vi "FRCts20_Backend_FGVDequeueDataReturn.vi"(6 "Engine_Refnums":T1, 7 "Operation":T4, 8 "error in (no error)":errorcluster) -> (0 "error out":errorcluster, 1 "Key":string, 2 "Message Value":string, 3 "Message Name":string, 4 "Engine_Refnums Out":T1)   [LabVIEW 2013, in "FRCts20_Backend_Engine.lvlib"]
doc: "Takes the AMC queues and lets us dequeue data. All it stores is the AMC queues."
uses:
  FRCts20_Backend_Engine.lvlib
  FRCts20_Backend_EngineRefnums.ctl
  INI_Accessor/FRCts20_Backend_INI Controller.lvclass
  Dependencies/AMC/_SubVIs/TypeDefs/Message Queue.ctl
  Dependencies/AMC/_SubVIs/TypeDefs/Message.ctl
  Dependencies/Keyed Array/KeyedArray.ctl
  <vilib>/addons/database/Connection.llb/Conn ObjectReference.ctl
  FRCts20_Backend_DequeueDataOperations.ctl
  Dependencies/AMC/AMC.lvlib
  Dependencies/Keyed Array/Tools_KeyedArray.lvlib
  <vilib>/addons/database/NI_Database_API.lvlib
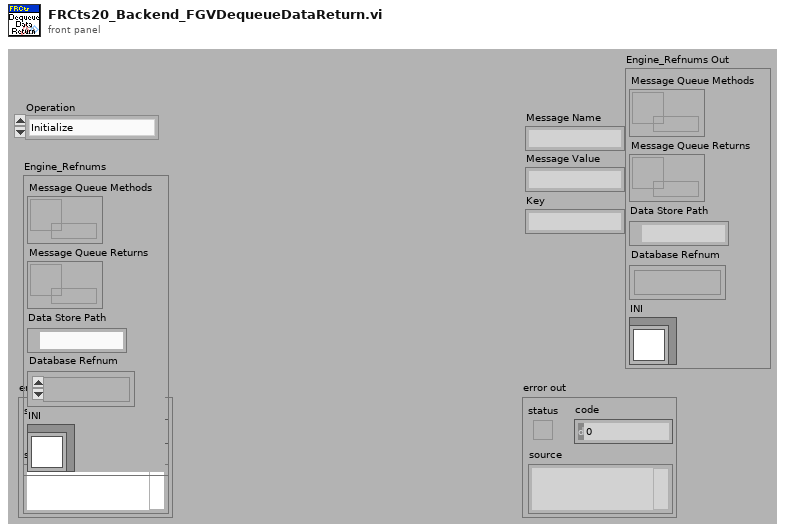
[diagram p1: front panel]
types:
  T1 = typedef "FRCts20_Backend_Engine.lvlib/FRCts20_Backend_EngineRefnums.ctl" = cluster{"Message Queue Methods":T2, "Message Queue Returns":T2, "Data Store Path":path, "Database Refnum":T3, "INI":refnum<class "FRCts20_Backend_INI Controller.lvclass">}
  T2 = typedef "AMC.lvlib/Message Queue.ctl" = refnum<queue>
  T3 = typedef "NI_Database_API.lvlib/Conn ObjectReference.ctl" = refnum<k1>
  T4 = typedef "FRCts20_Backend_Engine.lvlib/FRCts20_Backend_DequeueDataOperations.ctl" = enum16{"Initialize", "DequeueDataReturn", "GetQueues"}
  T5 = typedef "Tools_KeyedArray.lvlib/KeyedArray.ctl" = cluster{"keys":string[], "values":string[]}
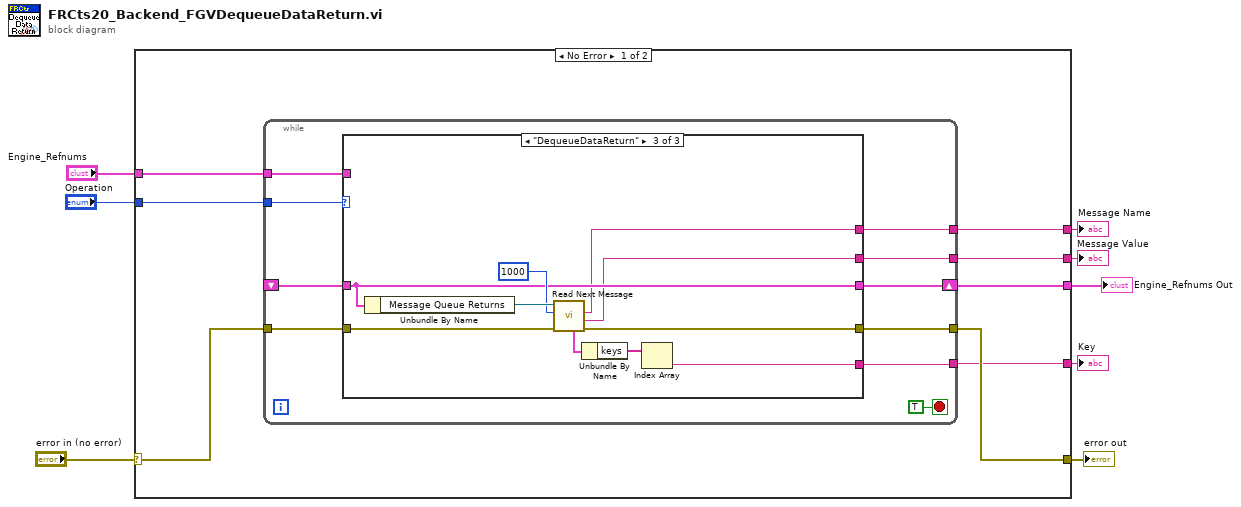
[diagram p0: block diagram]
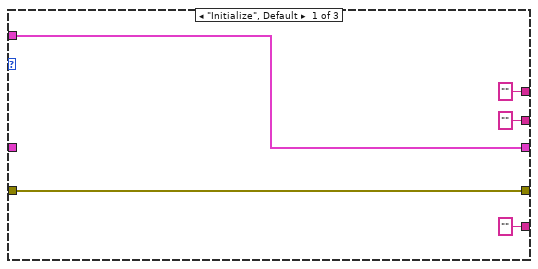
[diagram p2: hidden frame]
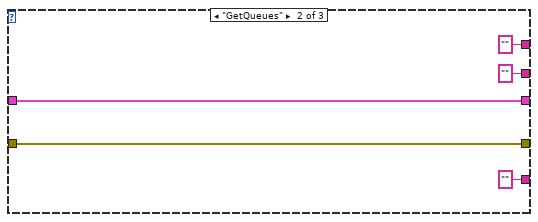
[diagram p3: hidden frame]
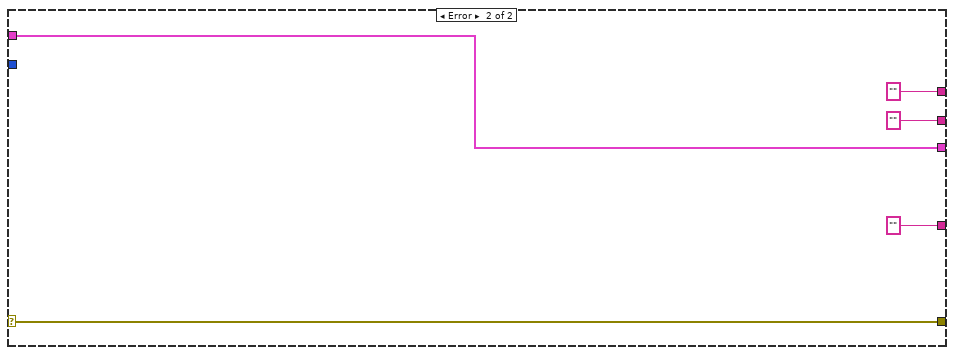
[diagram p4: hidden frame]
diagram:
  n1 = case shown="No Error" "error in (no error)" {
    selector: "error in (no error)" -> [w14 w51]
    tunnel: [w16 w51] -> w7
    tunnel: "Engine_Refnums" -> [w15 w47]
    tunnel: "Operation" -> [w13 _]
    tunnel: [w12 "" ("Message Name")] -> w4
    tunnel: [w11 "" ("Message Value")] -> w3
    tunnel: [w10 "" ("String")] -> w2
    tunnel: [w9 w47] -> w1
    frame No Error {
      n2 = while {
        tunnel: [w25] -> w16
        tunnel: w15 -> [w24]
        shift-right: [w23] -> w9
        shift-left: _ -> [w22]
        tunnel: w14 -> [w21]
        tunnel: w13 -> [w20]
        tunnel: [w19] -> w12
        tunnel: [w18] -> w11
        tunnel: [w17] -> w10
        stop <- TRUE stop-if-true
        n3 = case shown="\"DequeueDataReturn\"" w20 {
          tunnel: [w30 w36 w42] -> w25
          tunnel: w24 -> [w31 _ _]
          tunnel: [w31 w32 w43] -> w23
          tunnel: w22 -> [_ w32 w43]
          tunnel: w21 -> [w30 w36 w45]
          tunnel: ["" ("Message Name") "" ("Message Name") w41] -> w19
          tunnel: ["" ("Message Value") "" ("Message Value") w40] -> w18
          tunnel: ["" ("String") "" ("String") w37] -> w17
          frame "Initialize", Default {
          }
          frame "GetQueues" {
          }
          frame "DequeueDataReturn" {
            n4 = Unbundle By Name(w43) -> ("Message Queue Returns"=w46:T2)
            n5 = call "Read Next Message.vi"("error in (no error)"=w45, "timeout (1ms)"=1000, "Message Queue in"=w46) -> ("error out"=w42:errorcluster, "Message Value"=w40:string, "Message Name"=w41:string, "Message Attributes"=w39:T5)  [unwired: 2 in, 3 out]
            n6 = Unbundle By Name(w39) -> ("keys"=w38:string[])
            n7 = Index Array(array=w38) -> (element=w37:string)  [unwired: 1 in]
          }
        }
      }
    }
    frame Error {
    }
  }
  "error out" <- w7
  "Key" <- w2
  "Message Name" <- w4
  "Message Value" <- w3
  "Engine_Refnums Out" <- w1
